vi "Yellow to Red 1.vi"   [LabVIEW 2019]
uses:
  Global Var.vi
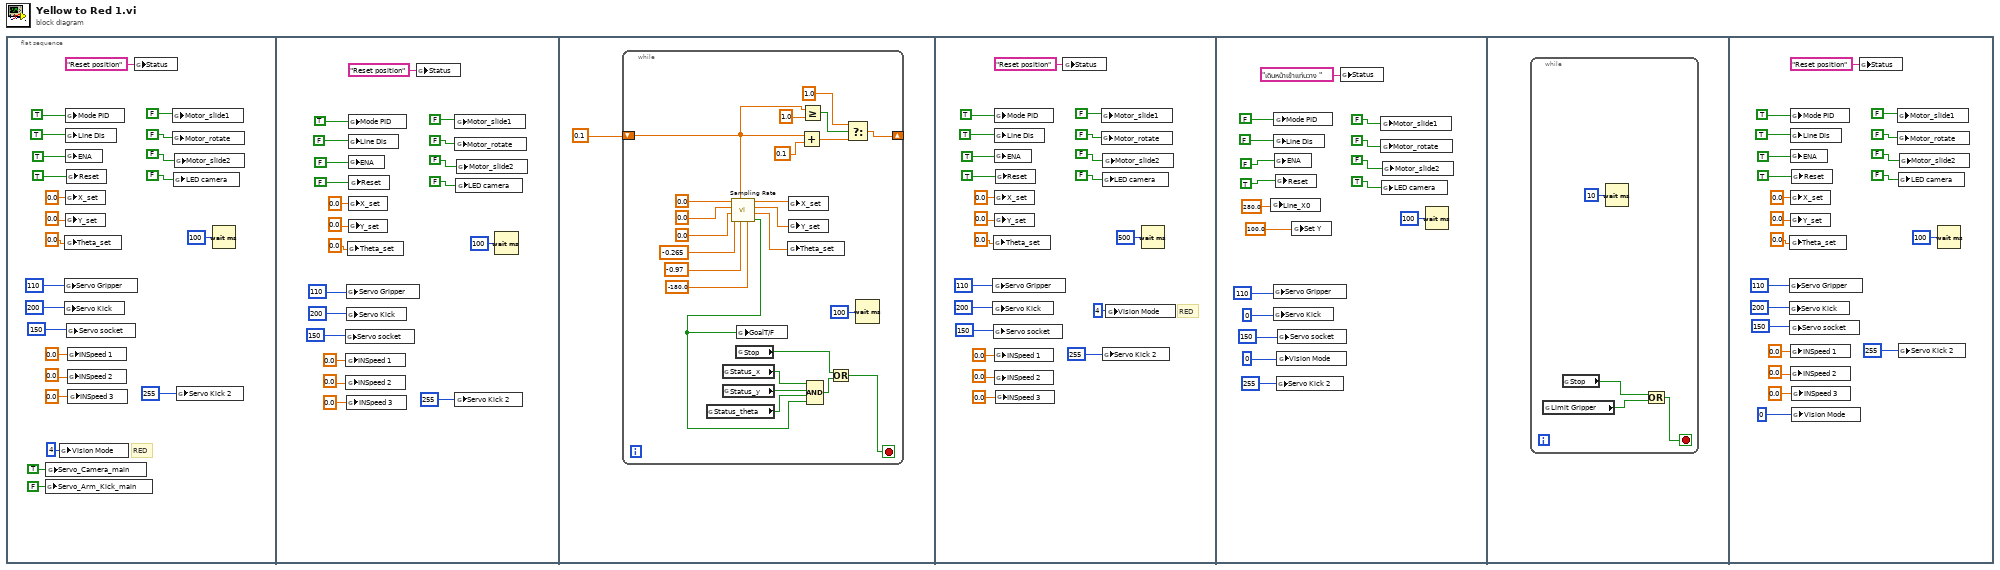
[diagram p0: block diagram]
diagram:
  n1 = flat-sequence {
    frame #0 {
      # "RED"
      n2 = global write "Global Var.vi" "Servo_Arm_Kick_main"(FALSE ("Mode PID")) -> ()
      n3 = global write "Global Var.vi" "Servo_Camera_main"(TRUE ("Mode PID")) -> ()
      n4 = global write "Global Var.vi" "Vision Mode"(i16 4 ("Vision Mode")) -> ()
      n5 = global write "Global Var.vi" "Servo Gripper"(u8 110 ("Servo Camera")) -> ()
      n6 = global write "Global Var.vi" "Servo Kick"(u8 200 ("Servo Camera")) -> ()
      n7 = global write "Global Var.vi" "Theta_set"(0.0 ("Theta_set")) -> ()
      n8 = global write "Global Var.vi" "Mode PID"(TRUE ("Mode PID")) -> ()
      n9 = global write "Global Var.vi" "Line Dis"(TRUE ("Mode PID")) -> ()
      n10 = global write "Global Var.vi" "ENA"(TRUE ("ENA")) -> ()
      n11 = global write "Global Var.vi" "X_set"(0.0 ("X_set")) -> ()
      n12 = global write "Global Var.vi" "Y_set"(0.0 ("Y_set")) -> ()
      n13 = global write "Global Var.vi" "Reset"(TRUE ("ENA")) -> ()
      n14 = global write "Global Var.vi" "Servo socket"(u8 150 ("Servo Camera")) -> ()
      n15 = global write "Global Var.vi" "INSpeed 1"(0.0 ("X_set")) -> ()
      n16 = global write "Global Var.vi" "INSpeed 2"(0.0 ("Y_set")) -> ()
      n17 = global write "Global Var.vi" "INSpeed 3"(0.0 ("Theta_set")) -> ()
      n18 = global write "Global Var.vi" "Status"("Reset position" ("Status")) -> ()
      n19 = global write "Global Var.vi" "Motor_slide1"(FALSE ("Mode PID")) -> ()
      n20 = global write "Global Var.vi" "Motor_rotate"(FALSE ("ENA")) -> ()
      n21 = global write "Global Var.vi" "LED camera"(FALSE ("LED camera")) -> ()
      n22 = global write "Global Var.vi" "Motor_slide2"(FALSE ("ENA")) -> ()
      n23 = global write "Global Var.vi" "Servo Kick 2"(u8 255 ("Servo Camera")) -> ()
      n24 = Wait (ms)(milliseconds to wait=u32 100) -> ()  [unwired: 1 out]
    }
    frame #1 {
      n25 = global write "Global Var.vi" "Servo socket"(u8 150 ("Servo Camera")) -> ()
      n26 = global write "Global Var.vi" "INSpeed 1"(0.0 ("X_set")) -> ()
      n27 = global write "Global Var.vi" "INSpeed 2"(0.0 ("Y_set")) -> ()
      n28 = global write "Global Var.vi" "Servo Gripper"(u8 110 ("Servo Camera")) -> ()
      n29 = global write "Global Var.vi" "Servo Kick"(u8 200 ("Servo Camera")) -> ()
      n30 = global write "Global Var.vi" "INSpeed 3"(0.0 ("Theta_set")) -> ()
      n31 = global write "Global Var.vi" "Theta_set"(0.0 ("Theta_set")) -> ()
      n32 = global write "Global Var.vi" "Mode PID"(TRUE ("Mode PID")) -> ()
      n33 = global write "Global Var.vi" "Line Dis"(FALSE ("Mode PID")) -> ()
      n34 = global write "Global Var.vi" "ENA"(FALSE ("ENA")) -> ()
      n35 = global write "Global Var.vi" "X_set"(0.0 ("X_set")) -> ()
      n36 = global write "Global Var.vi" "Y_set"(0.0 ("Y_set")) -> ()
      n37 = global write "Global Var.vi" "Reset"(FALSE ("ENA")) -> ()
      n38 = global write "Global Var.vi" "Status"("Reset position" ("Status")) -> ()
      n39 = global write "Global Var.vi" "Motor_slide1"(FALSE ("Mode PID")) -> ()
      n40 = global write "Global Var.vi" "Motor_rotate"(FALSE ("ENA")) -> ()
      n41 = global write "Global Var.vi" "Servo Kick 2"(u8 255 ("Servo Camera")) -> ()
      n42 = global write "Global Var.vi" "LED camera"(FALSE ("LED camera")) -> ()
      n43 = global write "Global Var.vi" "Motor_slide2"(FALSE ("ENA")) -> ()
      n44 = Wait (ms)(milliseconds to wait=u32 100) -> ()  [unwired: 1 out]
    }
    frame #2 {
      n45 = while {
        shift-right: [w47] -> _
        shift-left: 0.1 -> [w45]
        stop <- w64 stop-if-true
        n46 = global read "Global Var.vi" "Status_theta"() -> (w66:bool)
        n47 = global read "Global Var.vi" "Status_x"() -> (w67:bool)
        n48 = global read "Global Var.vi" "Status_y"() -> (w68:bool)
        n49 = call "Sampling Rate.vi"("input a1"=-180.0, "input y1"=-0.97, "T(0-1)"=w45, "input x1"=-0.265, "input a0"=0.0, "input y0"=0.0, "input x0"=0.0) -> ("GoalT/F"=w52:bool, "a_output"=w59:dbl, "y_output"=w60:dbl, "x_output"=w61:dbl)  [unwired: 1 in]
        n50 = global read "Global Var.vi" "Stop"() -> (w62:bool)
        n51 = global write "Global Var.vi" "GoalT/F"(w52) -> ()
        n52 = global write "Global Var.vi" "Theta_set"(w59) -> ()
        n53 = global write "Global Var.vi" "X_set"(w61) -> ()
        n54 = global write "Global Var.vi" "Y_set"(w60) -> ()
        n55 = Add(x=w45, y=0.1) -> (x+y=w50:dbl)
        n56 = Greater Or Equal?(x=w45, y=1.0) -> (x >= y?=w49:bool)
        n57 = Compound Arithmetic op=AND(w67, w68, w66, w52) -> (w63:bool)
        n58 = Or(x=w62, y=w63) -> (x .or. y?=w64:bool)
        n59 = Select(t=1.0, s=w49, f=w50) -> (s? t:f=w47:dbl)
        n60 = Wait (ms)(milliseconds to wait=u32 100) -> ()  [unwired: 1 out]
      }
    }
    frame #3 {
      # "RED"
      n61 = global write "Global Var.vi" "Servo Gripper"(u8 110 ("Servo Camera")) -> ()
      n62 = global write "Global Var.vi" "Servo Kick"(u8 200 ("Servo Camera")) -> ()
      n63 = global write "Global Var.vi" "Theta_set"(0.0 ("Theta_set")) -> ()
      n64 = global write "Global Var.vi" "Servo socket"(u8 150 ("Servo Camera")) -> ()
      n65 = global write "Global Var.vi" "Mode PID"(TRUE ("Mode PID")) -> ()
      n66 = global write "Global Var.vi" "Line Dis"(TRUE ("Mode PID")) -> ()
      n67 = global write "Global Var.vi" "ENA"(TRUE ("ENA")) -> ()
      n68 = global write "Global Var.vi" "X_set"(0.0 ("X_set")) -> ()
      n69 = global write "Global Var.vi" "Y_set"(0.0 ("Y_set")) -> ()
      n70 = global write "Global Var.vi" "INSpeed 1"(0.0 ("X_set")) -> ()
      n71 = global write "Global Var.vi" "INSpeed 2"(0.0 ("Y_set")) -> ()
      n72 = global write "Global Var.vi" "Reset"(TRUE ("ENA")) -> ()
      n73 = global write "Global Var.vi" "INSpeed 3"(0.0 ("Theta_set")) -> ()
      n74 = global write "Global Var.vi" "Status"("Reset position" ("Status")) -> ()
      n75 = global write "Global Var.vi" "Motor_slide1"(FALSE ("Mode PID")) -> ()
      n76 = global write "Global Var.vi" "Motor_rotate"(FALSE ("ENA")) -> ()
      n77 = global write "Global Var.vi" "LED camera"(FALSE ("LED camera")) -> ()
      n78 = global write "Global Var.vi" "Servo Kick 2"(u8 255 ("Servo Camera")) -> ()
      n79 = global write "Global Var.vi" "Motor_slide2"(FALSE ("ENA")) -> ()
      n80 = global write "Global Var.vi" "Vision Mode"(i16 4 ("Vision Mode")) -> ()
      n81 = Wait (ms)(milliseconds to wait=u32 500) -> ()  [unwired: 1 out]
    }
    frame #4 {
      n82 = global write "Global Var.vi" "Line_X0"(280.0 ("Y_set")) -> ()
      n83 = global write "Global Var.vi" "Servo Gripper"(u8 110 ("Servo Camera")) -> ()
      n84 = global write "Global Var.vi" "Servo Kick"(u8 0 ("Servo Camera")) -> ()
      n85 = global write "Global Var.vi" "Mode PID"(FALSE ("Mode PID")) -> ()
      n86 = global write "Global Var.vi" "Line Dis"(FALSE ("Mode PID")) -> ()
      n87 = global write "Global Var.vi" "ENA"(FALSE ("ENA")) -> ()
      n88 = global write "Global Var.vi" "Reset"(TRUE ("ENA")) -> ()
      n89 = global write "Global Var.vi" "Servo Kick 2"(u8 255 ("Servo Camera")) -> ()
      n90 = global write "Global Var.vi" "Vision Mode"(i16 0 ("Vision Mode")) -> ()
      n91 = global write "Global Var.vi" "Servo socket"(u8 150 ("Servo Camera")) -> ()
      n92 = global write "Global Var.vi" "Set Y"(100.0 ("Y_set")) -> ()
      n93 = global write "Global Var.vi" "Status"("เดินหน้าเข้าแท่นวาง " ("Status")) -> ()
      n94 = global write "Global Var.vi" "Motor_slide1"(FALSE ("Mode PID")) -> ()
      n95 = global write "Global Var.vi" "Motor_rotate"(FALSE ("ENA")) -> ()
      n96 = global write "Global Var.vi" "LED camera"(TRUE ("LED camera")) -> ()
      n97 = global write "Global Var.vi" "Motor_slide2"(FALSE ("ENA")) -> ()
      n98 = Wait (ms)(milliseconds to wait=u32 100) -> ()  [unwired: 1 out]
    }
    frame #5 {
      n99 = while {
        stop <- w109 stop-if-true
        n100 = global read "Global Var.vi" "Limit Gripper"() -> (w107:bool)
        n101 = global read "Global Var.vi" "Stop"() -> (w108:bool)
        n102 = Wait (ms)(milliseconds to wait=u32 10) -> ()  [unwired: 1 out]
        n103 = Or(x=w108, y=w107) -> (x .or. y?=w109:bool)
      }
    }
    frame #6 {
      n104 = global write "Global Var.vi" "Servo Gripper"(u8 110 ("Servo Camera")) -> ()
      n105 = global write "Global Var.vi" "Servo Kick"(u8 200 ("Servo Camera")) -> ()
      n106 = global write "Global Var.vi" "Theta_set"(0.0 ("Theta_set")) -> ()
      n107 = global write "Global Var.vi" "Servo socket"(u8 150 ("Servo Camera")) -> ()
      n108 = global write "Global Var.vi" "Mode PID"(TRUE ("Mode PID")) -> ()
      n109 = global write "Global Var.vi" "Line Dis"(TRUE ("Mode PID")) -> ()
      n110 = global write "Global Var.vi" "ENA"(TRUE ("ENA")) -> ()
      n111 = global write "Global Var.vi" "X_set"(0.0 ("X_set")) -> ()
      n112 = global write "Global Var.vi" "Y_set"(0.0 ("Y_set")) -> ()
      n113 = global write "Global Var.vi" "INSpeed 1"(0.0 ("X_set")) -> ()
      n114 = global write "Global Var.vi" "INSpeed 2"(0.0 ("Y_set")) -> ()
      n115 = global write "Global Var.vi" "Reset"(TRUE ("ENA")) -> ()
      n116 = global write "Global Var.vi" "INSpeed 3"(0.0 ("Theta_set")) -> ()
      n117 = global write "Global Var.vi" "Vision Mode"(i16 0 ("Vision Mode")) -> ()
      n118 = global write "Global Var.vi" "Status"("Reset position" ("Status")) -> ()
      n119 = global write "Global Var.vi" "Motor_slide1"(FALSE ("Mode PID")) -> ()
      n120 = global write "Global Var.vi" "Motor_rotate"(FALSE ("ENA")) -> ()
      n121 = global write "Global Var.vi" "LED camera"(FALSE ("LED camera")) -> ()
      n122 = global write "Global Var.vi" "Servo Kick 2"(u8 255 ("Servo Camera")) -> ()
      n123 = global write "Global Var.vi" "Motor_slide2"(FALSE ("ENA")) -> ()
      n124 = Wait (ms)(milliseconds to wait=u32 100) -> ()  [unwired: 1 out]
    }
  }
